vi "APTcontrol.vi"() -> ()   [LabVIEW 2013]
panel:
  out "Current position":sgl
  in  "stop":bool
  in  "Set position":sgl min=0 max=500
  out "error out":errorcluster
  in  "error in (no error)":errorcluster
  in  "MG17Piezo":refnum<k7>(container)
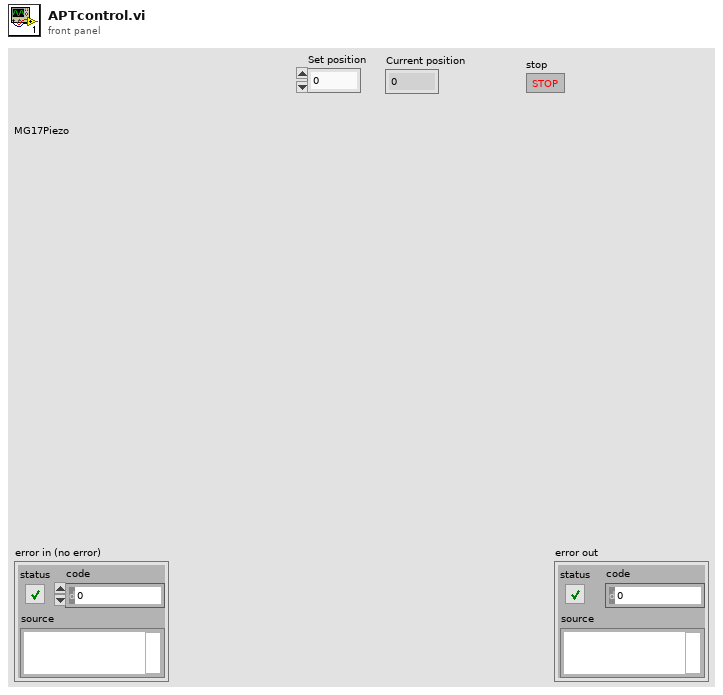
[diagram p1: front panel]
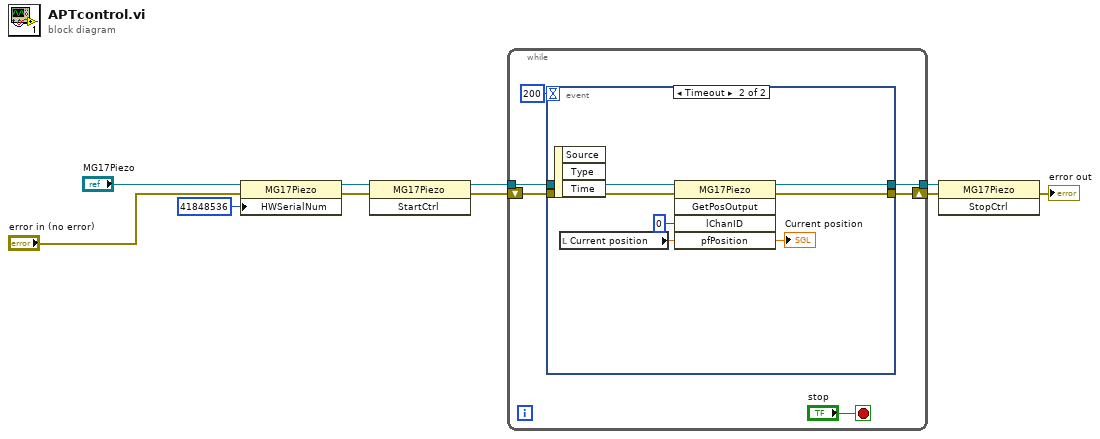
[diagram p0: block diagram]
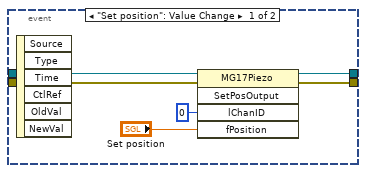
[diagram p2: hidden frame]
diagram:
  n1 = property class="MG17Piezo"(reference="MG17Piezo", error in="error in (no error)", "HWSerialNum"=41848536) -> (reference out=w8:refnum<k7>, error out=w7:errorcluster)
  n2 = invoke class="MG17Piezo" method="StartCtrl"(reference=w8, error in=w7) -> (reference out=w5:refnum<k7>, error out=w4:errorcluster)  [unwired: 1 in, 1 out]
  n3 = while {
    tunnel: [w15] -> w3
    tunnel: w5 -> [w16]
    shift-right: [w13] -> w2
    shift-left: w4 -> [w14]
    stop <- "stop" stop-if-true
    n4 = event shown="[1] Timeout" {
      selector: _ -> [_ _]
      dyn-events: _ -> [_ _]
      timeout: 200 -> [_ _]
      tunnel: w16 -> [w21 w27]
      tunnel: [w20 w28] -> w15
      tunnel: w14 -> [w19 w26]
      tunnel: [w18 w25] -> w13
      event "Set position": Value Change {
        n5 = event-data() -> ()  [unwired: 1 in, 6 out]
        n6 = invoke class="MG17Piezo" method="SetPosOutput"(reference=w21, error in=w19, "lChanID"=0, "fPosition"="Set position") -> (reference out=w20:refnum<k7>, error out=w18:errorcluster)  [unwired: 1 in, 3 out]
      }
      event Timeout {
        n7 = event-data() -> ()  [unwired: 1 in, 3 out]
        n8 = local read "Current position"() -> (w23:sgl)
        n9 = invoke class="MG17Piezo" method="GetPosOutput"(reference=w27, error in=w26, "lChanID"=0, "pfPosition"=w23) -> (reference out=w28:refnum<k7>, error out=w25:errorcluster, "pfPosition"=→"Current position":sgl)  [unwired: 1 in, 2 out]
      }
    }
  }
  n10 = invoke class="MG17Piezo" method="StopCtrl"(reference=w3, error in=w2) -> (error out=→"error out":errorcluster)  [unwired: 1 in, 2 out]
